vi "Scan Engine EtherCAT Master.vi"(8 "error in (no error)":errorcluster, 11 "Node Ptr":T1 format="%.0x") -> (0 "error out":errorcluster)   [LabVIEW 2016, in "Scan Engine Custom Device.lvlib"]
uses:
  Scan Engine Custom Device.lvlib
  <vilib>/NI Veristand/Custom Device API/Custom Device API.lvlib
  Globals/Property Strings.vi
  <vilib>/NI Veristand/Custom Device API/Get Item Property (U32).vi
  <vilib>/NI Veristand/Custom Device API/Set Item Property (U32).vi
  Globals/RT Globals.vi
  <vilib>/NI Veristand/Custom Device API/Custom Device Item Ref.ctl
panel:
  in  "SHDocVw.IWebBrowser2":refnum<k7>(container)
  in  "Cyclic Data Bandwidth (%)":u32=40 max=100
  in  "Add EtherCAT Slave":bool
  in  "Master ID":u32
  in  "Header":cluster{"Section Name":string}={"Section Name"="EtherCAT Master Settings"}
  in  "Name":string
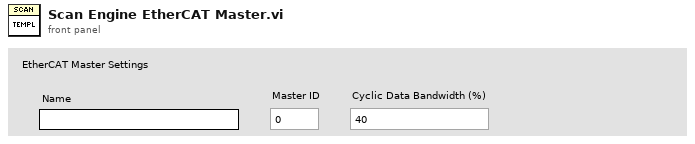
[diagram p1: front panel]
types:
  T1 = typedef "Custom Device API.lvlib/Custom Device Item Ref.ctl" = u64
  T2 = typedef "Custom Device API.lvlib/Custom Device Commands.ctl" = enum16{"Default", "Item renamed", "Shutdown", "Dynamic button pressed"}
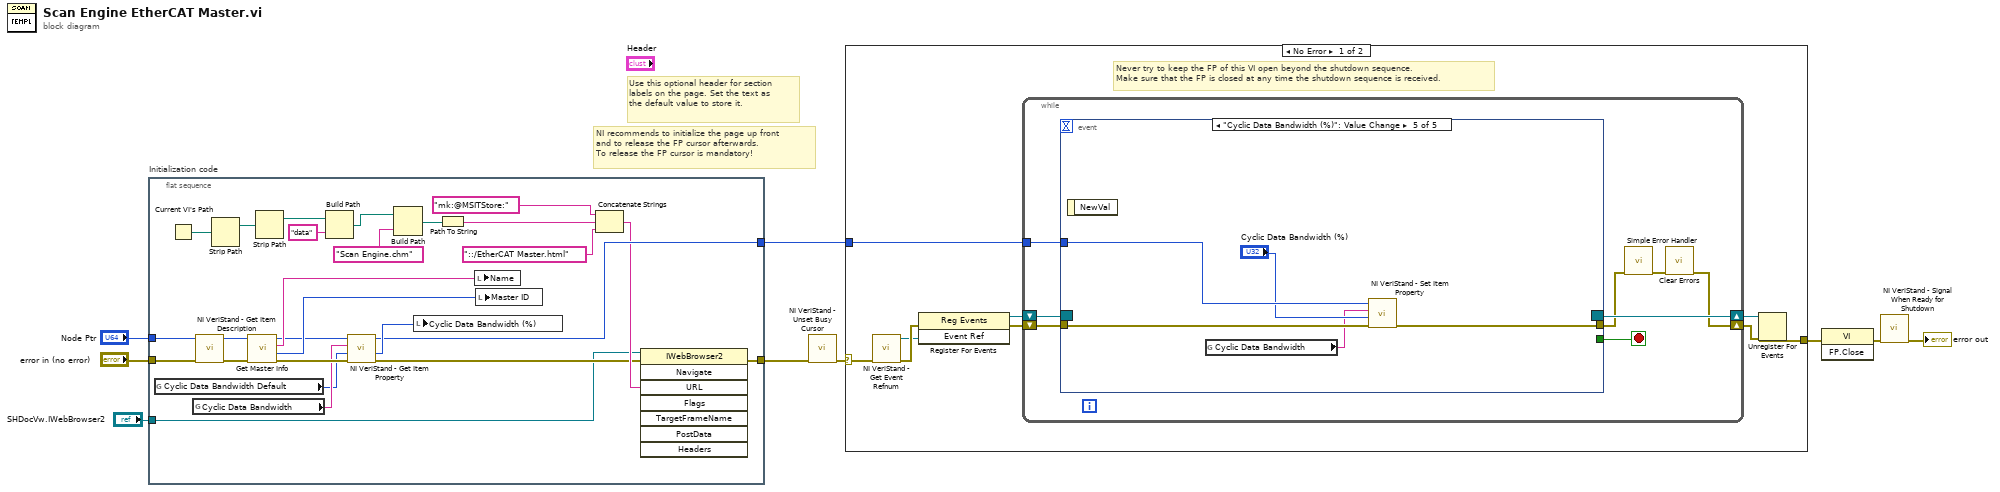
[diagram p0: block diagram]
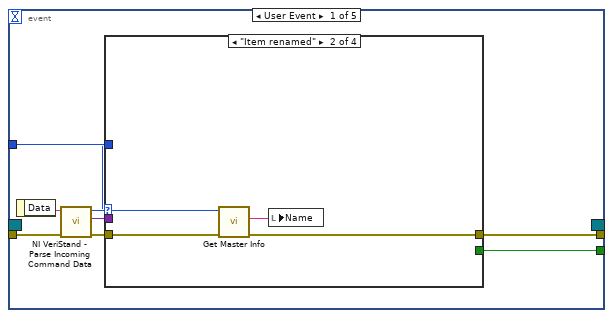
[diagram p2: hidden frame]
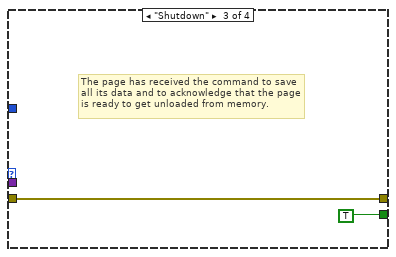
[diagram p4: hidden frame]
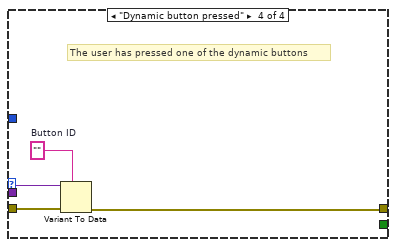
[diagram p5: hidden frame]
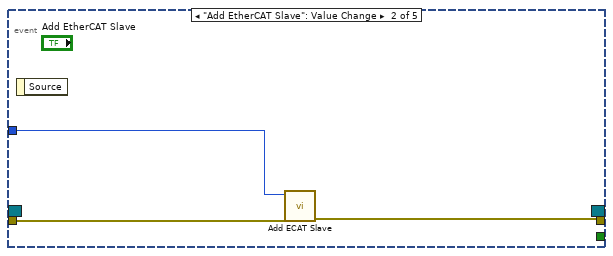
[diagram p6: hidden frame]
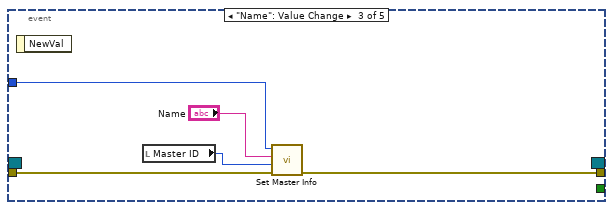
[diagram p7: hidden frame]
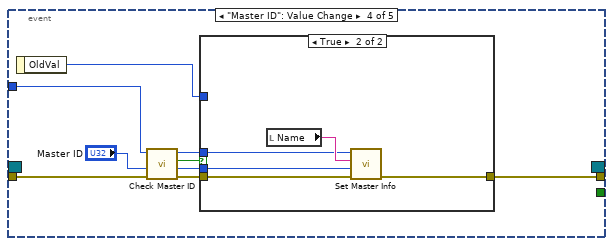
[diagram p8: hidden frame]
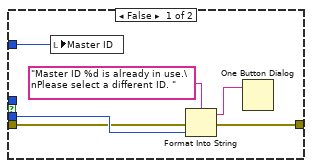
[diagram p9: hidden frame]
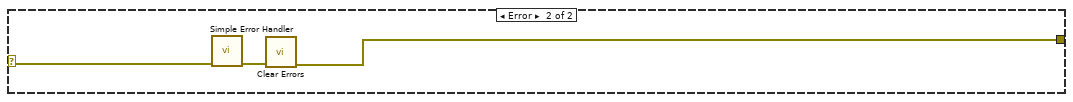
[diagram p10: hidden frame]
diagram:
  # "Use this optional header for section labels on the page. Set the text as the default value to store it."
  # "NI recommends to initialize the page up front\nand to release the FP cursor afterwards.\nTo release the FP cursor is mandatory!"
  n1 = flat-sequence "Initialization code" {
    tunnel: "error in (no error)" -> [w35]
    tunnel: "Node Ptr" -> [w34]
    tunnel: [w14] -> w5
    tunnel: [w25] -> w2
    tunnel: "SHDocVw.IWebBrowser2" -> [w11]
    frame #0 {
      n2 = global read "RT Globals.vi" "Cyclic Data Bandwidth Default"() -> (w10:u32)
      n3 = Current VI's Path() -> (path=w23:path)
      n4 = global read "Property Strings.vi" "Cyclic Data Bandwidth"() -> (w27:string)
      n5 = call <vilib>:"NI VeriStand - Get Item Description.vi"("error in (no error)"=w35, "Item Ref in"=w34) -> ("error out"=w32:errorcluster, "Item Ref out"=w33:T1)  [unwired: 8 out]
      n6 = Strip Path(path=w23) -> (stripped path=w22:path)  [unwired: 1 out]
      n7 = call "Get Master Info.vi"("error in (no error)"=w32, "Item Ref in"=w33) -> ("error out"=w28:errorcluster, "Master #"=w30:u32, "Master Name"=w31:string, "Item Ref out"=w29:T1)  [unwired: 6 in]
      n8 = Strip Path(path=w22) -> (stripped path=w17:path)  [unwired: 1 out]
      n9 = Build Path(base path=w17, name or relative path="data") -> (appended path=w16:path)
      n10 = call-poly <vilib>:"NI VeriStand - Get Item Property.vi"("error in (no error)"=w28, "Default Value"=w10, "Property Name"=w27, "Item Ref in"=w29) -> ("error out"=w12:errorcluster, "Value"=w26:u32, "Item Ref out"=w25:T1)  [unwired: 4 in, 1 out]
      n11 = Build Path(base path=w16, name or relative path="Scan Engine.chm") -> (appended path=w19:path)
      n12 = local write "Cyclic Data Bandwidth (%)"(w26) -> ()
      n13 = Path To String(path=w19) -> (string=w20:string)
      n14 = local write "Name"(w31) -> ()
      n15 = local write "Master ID"(w30) -> ()
      n16 = Concatenate Strings("mk:@MSITStore:" ("string"), w20, "::/EtherCAT Master.html" ("name or relative path")) -> (w13:string)
      n17 = invoke class="IWebBrowser2" method="Navigate"(reference=w11, error in=w12, "URL"=w13) -> (error out=w14:errorcluster)  [unwired: 5 in, 7 out]
    }
  }
  n18 = call <vilib>:"NI VeriStand - Unset Busy Cursor.vi"("error in (no error)"=w5) -> ("error out"=w4:errorcluster)  [unwired: 10 out]
  n19 = case shown="No Error" w4 {
    selector: w4 -> [w36 w107]
    tunnel: [w41 w105] -> w9
    tunnel: w2 -> [w37 _]
    frame No Error {
      # "Never try to keep the FP of this VI open beyond the shutdown sequence.\nMake sure that the FP is closed at any time the shutdown sequence is received."
      n20 = call <vilib>:"NI VeriStand - Get Event Refnum.vi"("error in (no error)"=w36) -> ("error out"=w44:errorcluster, "Event Ref"=w40:refnum<user-event>)  [unwired: 9 out]
      n21 = register-events(error in=w44, w40) -> (reference out=w38:refnum<event-registration>, error out=w39:errorcluster)  [unwired: 1 in]
      n22 = while {
        tunnel: w37 -> [w48]
        shift-right: [w45] -> w42
        shift-left: w39 -> [w51]
        shift-right: [w52] -> w43
        shift-left: w38 -> [w50]
        stop <- w49 stop-if-true
        n23 = event shown="[4] \"Cyclic Data Bandwidth (%)\": Value Change" {
          selector: w50 -> [_ _ _ _ _]
          dyn-events: [_ _ _ _ _] -> w52
          timeout: _ -> [_ _ _ _ _]
          tunnel: w51 -> [w60 w74 w79 w87 w104]
          tunnel: [w56 _ _ _ _] -> w49
          tunnel: [w55 w72 w78 w88 w100] -> w47
          tunnel: w48 -> [w54 w73 w76 w85 w103]
          event User Event {
            n24 = event-data() -> ("Data"=w59:string)  [unwired: 1 out]
            n25 = call <vilib>:"NI VeriStand - Parse Incoming Command Data.vi"("error in (no error)"=w60, "Incoming data"=w59) -> ("error out"=w58:errorcluster, "Outgoing data"=w53:variant, "Action"=w57:T2)  [unwired: 7 out]
            n26 = case shown="\"Item renamed\"" w57 {
              tunnel: w58 -> [w61 w64 w66 w71]
              tunnel: [_ _ TRUE _] -> w56
              tunnel: [w61 w62 w66 w68] -> w55
              tunnel: w54 -> [_ w65 _ _]
              tunnel: w53 -> [_ _ _ w70]
              frame "Default", Default {
              }
              frame "Item renamed" {
                n27 = call "Get Master Info.vi"("error in (no error)"=w64, "Item Ref in"=w65) -> ("error out"=w62:errorcluster, "Master Name"=w63:string)  [unwired: 6 in, 2 out]
                n28 = local write "Name"(w63) -> ()
              }
              frame "Shutdown" {
                # "The page has received the command to save all its data and to acknowledge that the page is ready to get unloaded from memory."
              }
              frame "Dynamic button pressed" {
                w69 = ""  # Button ID
                # "The user has pressed one of the dynamic buttons"
                n29 = Variant To Data(error in=w71, type=w69, Variant=w70) -> (error out=w68:errorcluster)  [unwired: 1 out]
              }
            }
          }
          event "Add EtherCAT Slave": Value Change {
            n30 = event-data() -> ()  [unwired: 2 out]
            n31 = call "Add ECAT Slave.vi"("error in (no error)"=w74, "ECAT Master Ref in"=w73) -> ("error out"=w72:errorcluster)  [unwired: 8 in, 1 out]
          }
          event "Name": Value Change {
            n32 = event-data() -> ()  [unwired: 2 out]
            n33 = local read "Master ID"() -> (w75:u32)
            n34 = call "Set Master Info.vi"("error in (no error)"=w79, "Master #"=w75, "Master Name"="Name", "Item Ref in"=w76) -> ("error out"=w78:errorcluster)  [unwired: 6 in, 1 out]
          }
          event "Master ID": Value Change {
            n35 = event-data() -> ("OldVal"=w80:u32)  [unwired: 1 out]
            n36 = call "Check Master ID.vi"("error in (no error)"=w87, "Master ID in"="Master ID", "Item Ref in"=w85) -> ("error out"=w86:errorcluster, "Master ID out"=w82:u32, "Available?"=w81:bool, "Item Ref out"=w84:T1)  [unwired: 5 in]
            n37 = case shown="True" w81 {
              tunnel: [w90 w99] -> w88
              tunnel: w86 -> [w91 w97]
              tunnel: w84 -> [_ w96]
              tunnel: w82 -> [w93 w95]
              tunnel: w80 -> [w89 _]
              frame False {
                n38 = local write "Master ID"(w89) -> ()
                n39 = Format Into String(format string="Master ID %d is already in use.\nPlease select a different ID. ", error in=w91, w93) -> (resulting string=w92:string, error out=w90:errorcluster)  [unwired: 1 in]
                n40 = One Button Dialog(message=w92) -> ()  [unwired: 1 in, 1 out]
              }
              frame True {
                n41 = local read "Name"() -> (w98:string)
                n42 = call "Set Master Info.vi"("error in (no error)"=w97, "Master #"=w95, "Master Name"=w98, "Item Ref in"=w96) -> ("error out"=w99:errorcluster)  [unwired: 6 in, 1 out]
              }
            }
          }
          event "Cyclic Data Bandwidth (%)": Value Change {
            n43 = event-data() -> ()  [unwired: 2 out]
            n44 = global read "Property Strings.vi" "Cyclic Data Bandwidth"() -> (w101:string)
            n45 = call-poly <vilib>:"NI VeriStand - Set Item Property.vi"("error in (no error)"=w104, "Value"="Cyclic Data Bandwidth (%)", "Property Name"=w101, "Item Ref in"=w103) -> ("error out"=w100:errorcluster)  [unwired: 5 in, 2 out]
          }
        }
        n46 = call <vilib>:"Simple Error Handler.vi"("error in (no error)"=w47) -> ("error out"=w46:errorcluster)  [unwired: 1 in, 7 out]
        n47 = call <vilib>:"Clear Errors.vi"("error in (no error)"=w46) -> ("error out"=w45:errorcluster)  [unwired: 1 in, 5 out]
      }
      n48 = Unregister For Events(event registration refnum=w43, error in=w42) -> (error out=w41:errorcluster)
    }
    frame Error {
      n49 = call <vilib>:"Simple Error Handler.vi"("error in (no error)"=w107) -> ("error out"=w106:errorcluster)  [unwired: 1 in, 7 out]
      n50 = call <vilib>:"Clear Errors.vi"("error in (no error)"=w106) -> ("error out"=w105:errorcluster)  [unwired: 1 in, 5 out]
    }
  }
  n51 = invoke class="VI" method="FP.Close"(error in=w9) -> (error out=w8:errorcluster)  [unwired: 2 in, 2 out]
  n52 = call <vilib>:"NI VeriStand - Signal When Ready for Shutdown.vi"("error in (no error)"=w8) -> ("error out"=→"error out":errorcluster)  [unwired: 10 out]
